vi "PassBestRobotRole.vi"(5 "Robot":refnum<class "Robot.lvclass">, 7 "first call":bool, 8 "error in (no error)":errorcluster, 9 "Tactic index in":i32, 10 "Game in":refnum<class "Game.lvclass">, 11 "PassBestRobotRole in":refnum<class "PassBestRobotRole.lvclass">) -> (0 "error out":errorcluster, 1 "tactic index":i32, 2 "Robot out":refnum<class "Robot.lvclass">, 3 "PassBestRobotRole out":refnum<class "PassBestRobotRole.lvclass">, 4 "Game out":refnum<class "Game.lvclass">)   [LabVIEW 2023, in "PassBestRobotRole.lvclass"]
uses:
  PassBestRobotRole.lvclass
  C:/Users/lucio/Desktop/roboime/SSL_AI/Role_class/Role.lvclass
  Game_class/Game.lvclass
  Robot_class/Robot.lvclass
  Role_class/Role.lvclass/Role.ctl
  KickToBestRobotTactic_class/KickTOBestRobotTacticStatesEnum.ctl
  KickToBestRobotTactic_class/KickToBestRobotTactic.lvclass/KickToBestRobotTactic.ctl
  KickToBestRobotTactic_class/Read States.vi
  Role_class/Read Tacticbook.vi
  Role_class/Write Tacticbook.vi
  Role_class/Write tactic_index.vi
  Tacticbook_class/Tacticbook.lvclass
  KickToBestRobotTactic_class/KickToBestRobotTactic.lvclass
  5RobotsTactic_class/5RobotsTactic.lvclass
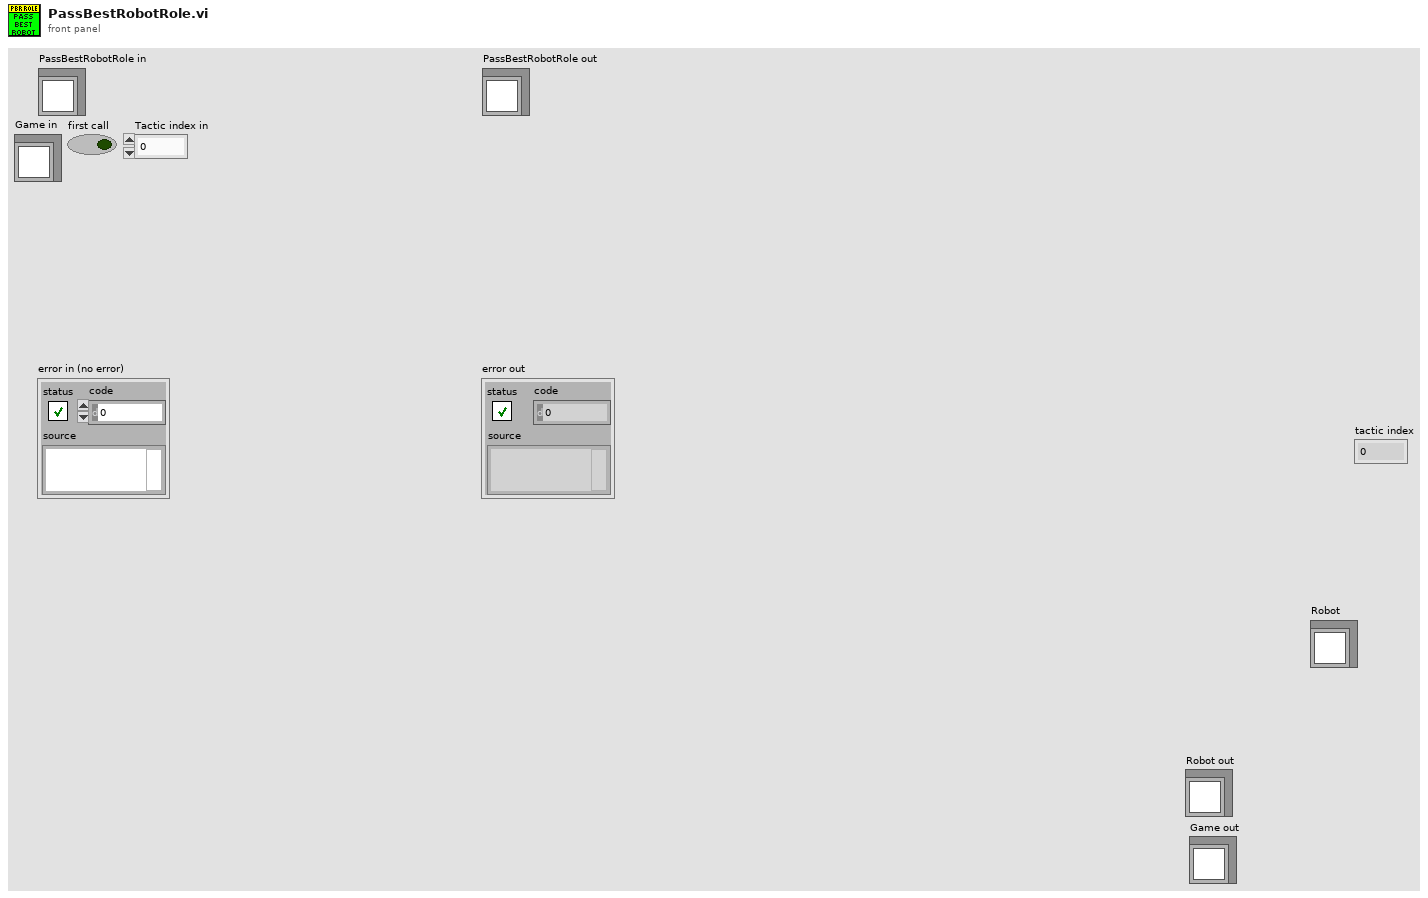
[diagram p1: front panel]
types:
  T1 = typedef "KickToBestRobotTactic.lvclass/KickTOBestRobotTacticStatesEnum.ctl" = enum16{"WaitToPass", "Pass", "Exit"}
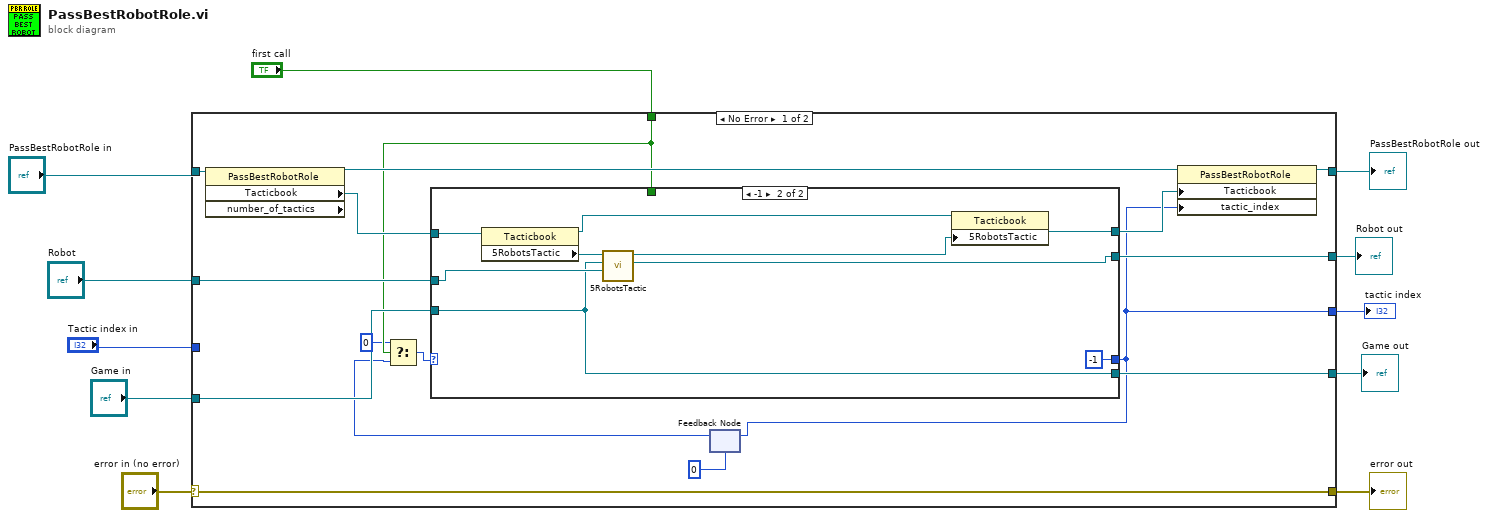
[diagram p0: block diagram]
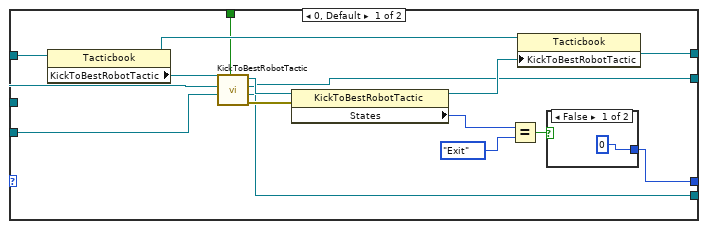
[diagram p2: hidden frame]
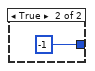
[diagram p3: hidden frame]
diagram:
  n1 = case shown="No Error" "error in (no error)" {
    selector: "error in (no error)" -> [w27 w58]
    tunnel: [w27 w58] -> w3
    tunnel: [w25 w57] -> w11
    tunnel: "PassBestRobotRole in" -> [w26 w57]
    tunnel: "Robot" -> [w19 w56]
    tunnel: [w22 w56] -> w6
    tunnel: [w18 w55] -> w4
    tunnel: "Game in" -> [w20 w55]
    tunnel: [w16 _] -> w5
    tunnel: "Tactic index in" -> [_ _]
    tunnel: "first call" -> [w13 _]
    frame No Error {
      n2 = property class="PassBestRobotRole" props=["Tacticbook", "number_of_tactics"](reference=w26) -> (reference out=w24:refnum<class "PassBestRobotRole.lvclass">, "Tacticbook"=w23:refnum<class "Tacticbook.lvclass">)  [unwired: 1 in, 2 out]
      n3 = feedback #1(0) -> (w15:i32)
      n4 = Select(t=0, s=w13, f=w15) -> (s? t:f=w14:i32)
      n5 = case shown="-1" w14 {
        tunnel: [w37 -1] -> w16
        tunnel: w23 -> [w43 w54]
        tunnel: w19 -> [w35 w50]
        tunnel: [w31 w48] -> w22
        tunnel: [w40 w52] -> w21
        tunnel: w20 -> [w34 w47]
        tunnel: w13 -> [w30 _]
        tunnel: [w29 w47] -> w18
        frame 0, Default {
          n6 = property class="Tacticbook"(reference=w43) -> (reference out=w42:refnum<class "Tacticbook.lvclass">, "KickToBestRobotTactic"=w36:refnum<class "KickToBestRobotTactic.lvclass">)  [unwired: 1 in, 1 out]
          n7 = call-dynamic "KickToBestRobotTactic.vi"("first call"=w30, "Game in"=w34, "Robot"=w35, "KickToBestRobotTactic in"=w36) -> ("error out"=w33:errorcluster, "Game out"=w29:refnum<class "Game.lvclass">, "Robot out"=w31:refnum<class "Robot.lvclass">, "KickToBestRobotTactic out"=w32:refnum<class "KickToBestRobotTactic.lvclass">)  [unwired: 4 in]
          n8 = property class="KickToBestRobotTactic"(reference=w32, error in=w33) -> (reference out=w41:refnum<class "KickToBestRobotTactic.lvclass">, "States"=w38:T1)  [unwired: 1 out]
          n9 = Equal?(x=w38, y=KickTOBestRobotTacticStatesEnum."Exit") -> (x = y?=w39:bool)
          n10 = property class="Tacticbook"(reference=w42, "KickToBestRobotTactic"=w41) -> (reference out=w40:refnum<class "Tacticbook.lvclass">)  [unwired: 1 in, 1 out]
          n11 = case shown="False" w39 {
            tunnel: [0 -1] -> w37
            frame False {
            }
            frame True {
            }
          }
        }
        frame -1 {
          n12 = property class="Tacticbook"(reference=w54) -> (reference out=w53:refnum<class "Tacticbook.lvclass">, "5RobotsTactic"=w51:refnum<class "5RobotsTactic.lvclass">)  [unwired: 1 in, 1 out]
          n13 = call "5RobotsTactic.vi"("Robot In"=w50, "Game in"=w47, "5RobotsTactic in"=w51) -> ("Robot out"=w48:refnum<class "Robot.lvclass">, "5RobotsTactic out"=w49:refnum<class "5RobotsTactic.lvclass">)  [unwired: 6 in, 1 out]
          n14 = property class="Tacticbook"(reference=w53, "5RobotsTactic"=w49) -> (reference out=w52:refnum<class "Tacticbook.lvclass">)  [unwired: 1 in, 1 out]
        }
      }
      n15 = feedback-in #1(w16) -> ()
      n16 = property class="PassBestRobotRole"(reference=w24, "Tacticbook"=w21, "tactic_index"=w16) -> (reference out=w25:refnum<class "PassBestRobotRole.lvclass">)  [unwired: 1 in, 1 out]
    }
    frame Error {
    }
  }
  "error out" <- w3
  "PassBestRobotRole out" <- w11
  "Robot out" <- w6
  "Game out" <- w4
  "tactic index" <- w5
